vi "AddFacesToTrack.vi"(8 "error in (no error)":errorcluster, 9 "Faces":T3[](array[typedef]) {"Rotation" format="%.2f"; "Left" scale=0.0..1024.0; "Right" scale=0.0..1024.0}, 10 "Image (duplicate) in":T2, 11 "Refnum in":T1) -> (0 "error out":errorcluster, 2 "Image (duplicate) out":T2, 3 "Refnum out":T1)   [LabVIEW 2019]
uses:
  <vilib>/vision/Image Controls.llb/IMAQ Image.ctl
  <vilib>/vision/Tracking.llb/IMAQ Object Tracking Session.ctl
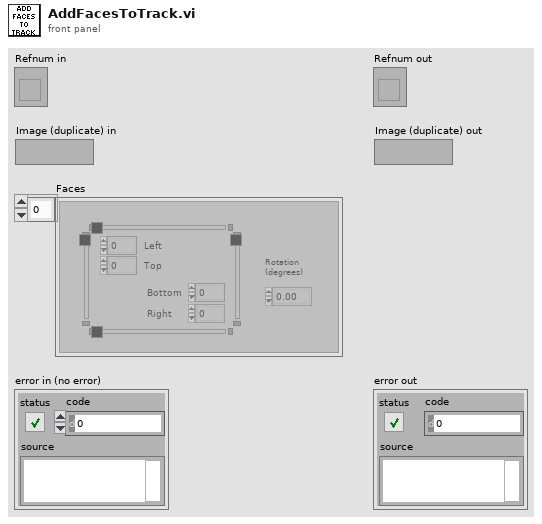
[diagram p1: front panel]
types:
  T1 = typedef "IMAQ Object Tracking Session.ctl" = refnum<k20>
  T2 = typedef "IMAQ Image.ctl" = refnum<image>
  T3 = typedef "IMAQ Rectangle" = cluster{"Left":i32, "Top":i32, "Right":i32, "Bottom":i32, "Rotation":dbl}
  T4 = typedef "ROI Descriptor" = cluster{"Global Rectangle":i32[], "Contours":cluster{"ID":enum32{"External", "Internal"}, "Type":u32, "Coordinates":i32[]}[]}
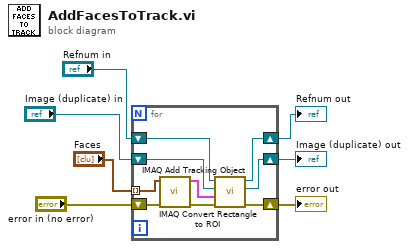
[diagram p0: block diagram]
diagram:
  n1 = for {
    shift-right: [w14] -> w5
    shift-left: "Refnum in" -> [w15]
    shift-right: [w10] -> w3
    shift-left: "error in (no error)" -> [w11]
    shift-right: [w9] -> w6
    shift-left: "Image (duplicate) in" -> [w16]
    tunnel: "Faces" -> [w8] mode=indexing
    n2 = call "IMAQ Convert Rectangle to ROI"("error in (no error)"=w11, "Rectangle"=w8) -> ("error out"=w12:errorcluster, "ROI Descriptor"=w13:T4)  [unwired: 7 in]
    n3 = call "IMAQ Add Tracking Object"("error in (no error)"=w12, "ROI Descriptor"=w13, "Image"=w16, "Object Tracking Session In"=w15) -> ("error out"=w10:errorcluster, "Image (duplicate)"=w9:T2, "Object Tracking Session Out"=w14:T1)  [unwired: 1 in, 4 out]
  }
  "Image (duplicate) out" <- w6
  "Refnum out" <- w5
  "error out" <- w3
